vi "Send Update Door Buttons.vi"(7 "Message Priority (Normal)":T2=enum."Normal", 8 "error in (no error)":errorcluster, 10 "Door Buttons":T1, 11 "Message Enqueuer":refnum<class "Message Enqueuer.lvclass">) -> (0 "error out":errorcluster, 3 "Message Enqueuer out":refnum<class "Message Enqueuer.lvclass">)   [LabVIEW 2022 SP3, in "Sim User Console Actor.lvlib" / "Update Door Buttons Msg.lvclass"]
doc: "This VI sends the message to an actor."
uses:
  Update Door Buttons Msg.lvclass
  <vilib>/ActorFramework/Message Enqueuer/Message Enqueuer.lvclass
  <vilib>/ActorFramework/Message Enqueuer/Message Priority.ctl
  Elevator Controller Actor/Door Buttons.ctl
  C:/Program Files/National Instruments/LabVIEW 2022/vi.lib/ActorFramework/Message/Message.lvclass
  Update Door Buttons Msg.lvclass/Update Door Buttons Msg.ctl
  <vilib>/ActorFramework/Message Enqueuer/Message Enqueuer.lvclass/Message Enqueuer.ctl
  <vilib>/ActorFramework/Message Priority Queue/Priority Enqueue.vi
  C:/Workspace/CLA/Elevator AF_2022_2nd/Sim User Console Actor/Sim User Console Actor Messages/Update Door Buttons Msg/Update Door Buttons Msg.lvclass
  Elevator Controller Actor/Sim User Console Actor.lvclass
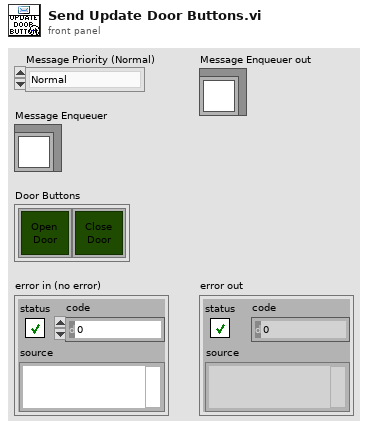
[diagram p1: front panel]
types:
  T1 = typedef "Sim User Console Actor.lvlib/Sim User Console Actor.lvclass/Door Buttons.ctl" = cluster{"Open Door":bool, "Close Door":bool}
  T2 = typedef "Actor Framework.lvlib/Message Enqueuer.lvclass/Message Priority.ctl" = enum16{"Low", "Normal", "High"}
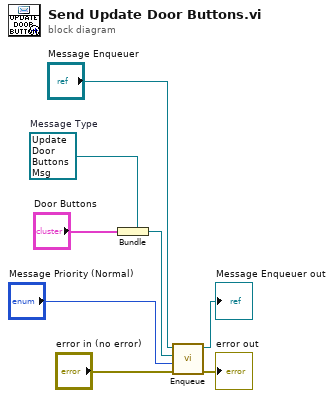
[diagram p0: block diagram]
diagram:
  w5 = refnum<class "Update Door Buttons Msg.lvclass"> refnum  # Message Type
  n1 = Bundle(cluster=w5, "Door Buttons") -> (w4:refnum<class "Update Door Buttons Msg.lvclass">)
  n2 = call <vilib>:"Enqueue.vi"("error in (no error)"="error in (no error)", "Message Priority (Normal)"="Message Priority (Normal)", "Message"=w4, "Message Enqueuer in"="Message Enqueuer") -> ("error out"=→"error out":errorcluster, "Message Enqueuer in"=→"Message Enqueuer out":refnum<class "Message Enqueuer.lvclass">)  [unwired: 6 in]
